vi "Write LAYER.vi"(8 "error in (no error)":errorcluster, 10 "LAYER":i16, 11 "Geometric in":refnum<class "Geometric.lvclass">) -> (0 "error out":errorcluster, 3 "Geometric out":refnum<class "Geometric.lvclass">)   [LabVIEW 2019, in "Geometric.lvclass"]
uses:
  Geometric.lvclass
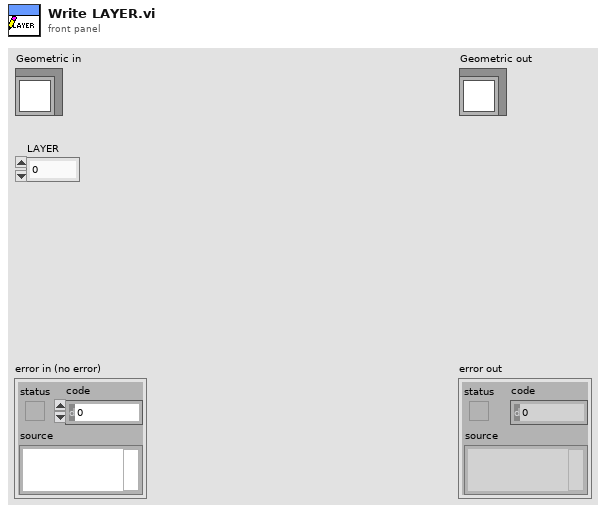
[diagram p1: front panel]
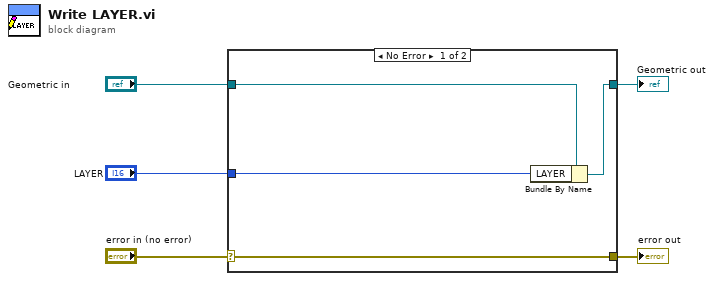
[diagram p0: block diagram]
diagram:
  n1 = case shown="No Error" "error in (no error)" {
    selector: "error in (no error)" -> [w9 w10]
    tunnel: [w9 w10] -> w4
    tunnel: [w7 w11] -> w2
    tunnel: "Geometric in" -> [w8 w11]
    tunnel: "LAYER" -> [w6 _]
    frame No Error {
      n2 = Bundle By Name(cluster=w8, "LAYER"=w6) -> (w7:refnum<class "Geometric.lvclass">)
    }
    frame Error {
    }
  }
  "error out" <- w4
  "Geometric out" <- w2
